vi "GlobalStop.vi"() -> ()   [LabVIEW 2011]
panel:
  in  "gSTOP":bool
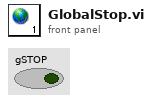
[diagram p1: front panel]
diagram:
